vi "isVisible.vi"(8 "Error In":errorcluster, 11 "QWinThumbnailToolButton In":refnum<class "QWinThumbnailToolButton.lvclass">) -> (0 "Error Out":errorcluster, 2 "Value":bool, 3 "QWinThumbnailToolButton Out":refnum<class "QWinThumbnailToolButton.lvclass">)   [LabVIEW 2014, in "QWinThumbnailToolButton.lvclass"]
doc: "LabVIEW-specific documentation is not yet available. See <b>https://doc.qt.io/qt-5/qwinthumbnailtoolbutton.html#isVisible</b>"
uses:
  QWinThumbnailToolButton.lvclass
  LQ Core/LQIdentity/LQIdentity.lvclass/LQIdentity.ctl
  LQ Core/LQ Core.lvlib
  LQ Core/LQIdentity/LQIdentity.lvclass
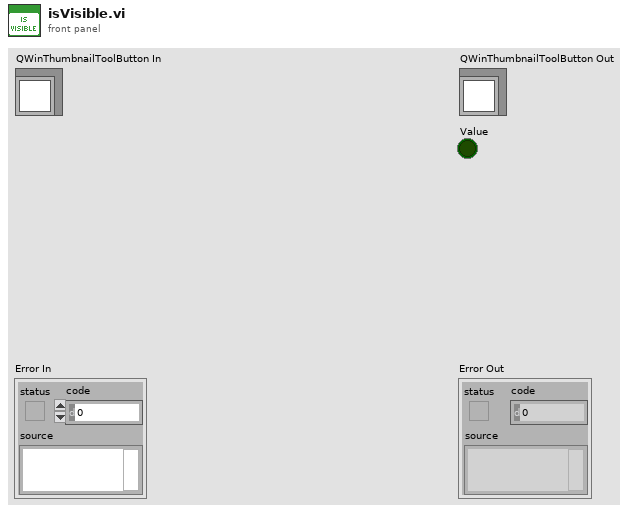
[diagram p1: front panel]
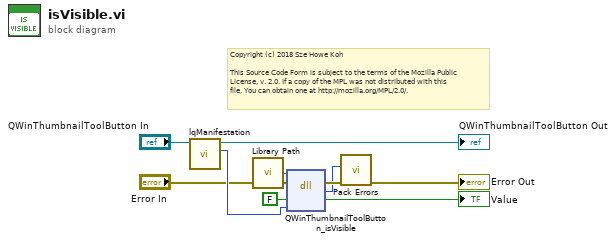
[diagram p0: block diagram]
diagram:
  # "Copyright (c) 2018 Sze Howe Koh\n\nThis Source Code Form is subject to the terms of the Mozilla Public\nLicense, v. 2.0. If a copy of the MPL was not distributed with this\nfile, You can obtain one at http://mozilla.org/MPL/2.0/."
  n1 = call "lqManifestation.vi"("LQIdentity in"="QWinThumbnailToolButton In") -> ("Manifestation"=w5:u64, "LQIdentity out"=→"QWinThumbnailToolButton Out":refnum<class "QWinThumbnailToolButton.lvclass">)  [unwired: 9 in]
  n2 = call "Library Path.vi"() -> ("Library Path"=w6:path)
  n3 = dll-call lib="?" fn="QWinThumbnailToolButton_isVisible"(path in=w6, error in="Error In", "_retVal"=FALSE, "_instance"=w5) -> (error out=w3:errorcluster, w1:i32, "_retVal"=→"Value":bool)  [unwired: 2 in, 1 out]
  n4 = call "Pack Errors.vi"("Error In"=w3, "Error Code"=w1) -> ("Error Out"=→"Error Out":errorcluster)  [unwired: 9 in]
